vi "RT (Testing).vi"() -> ()   [LabVIEW 2015]
uses:
  <vilib>/FPGAPlugInAG/sbRIO-9626/niLvFpga_Open_sbRIO-9626.vi
  <vilib>/rvi/interface/common/dynamic/niFpgaDynamicAddResources.vi
  <vilib>/Utility/error.llb/Error Cluster From Error Code.vi
  <vilib>/rvi/errors/niLvFpgaAdjustHostInterfaceError.vi
  <vilib>/FPGAPlugInAG/Dynamic/niLvFpga_Close_Dynamic.vi
  <vilib>/rvi/interface/nirviOpenFPGA/nirviOpenFPGA.xnode
  FPGA/Bitfiles/myPAM_FPGA_FPGA(TopLevel)_6BC50j0dlkU.lvbitx
  FPGA/FPGA (Top Level).vi
  <vilib>/rvi/interface/nirviReadWriteControl/nirviReadWriteControl.xnode
  <vilib>/rvi/interface/nirviCloseFPGA/nirviCloseFPGA.xnode
  NiFpgaLv.dll
  <vilib>/rvi/interface/Simulation/niFpgaSimulationCallBeginRW.vi
panel:
  out "LINK2_DRIVE_STATUS":T1(ring)
  out "LINK1_DRIVE_STATUS":T1(ring)
  in  "LINK2_DEMAND_PWM":i16(slide) scale=-375.0..375.0
  in  "LINK1_DEMAND_PWM":i16(slide) scale=-525.0..525.0
  in  "LINK2_DRIVE_ENABLED":bool
  in  "LINK1_DRIVE_ENABLED":bool
  in  "Stop Button":bool
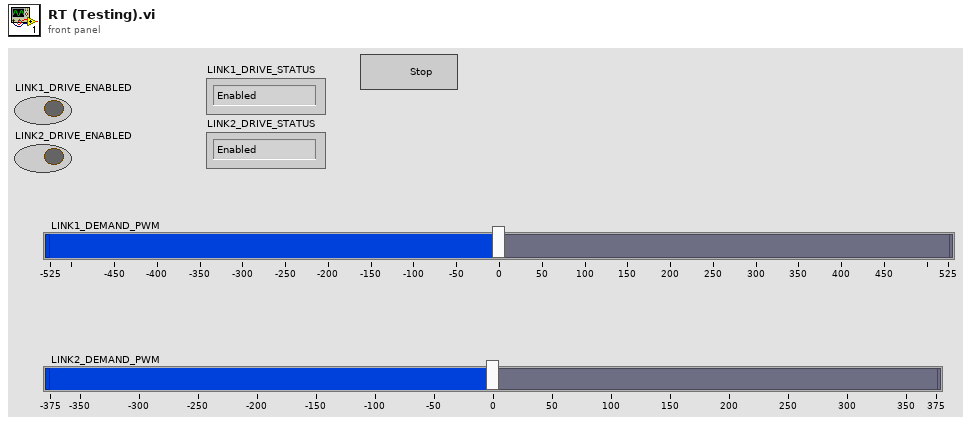
[diagram p1: front panel]
types:
  T1 = enum8{"Enabled", "Disabled", "Disabled by Drive Fault", "Disabled by Temp. Fault", "Disabled by E-Stop", "Unknown"}
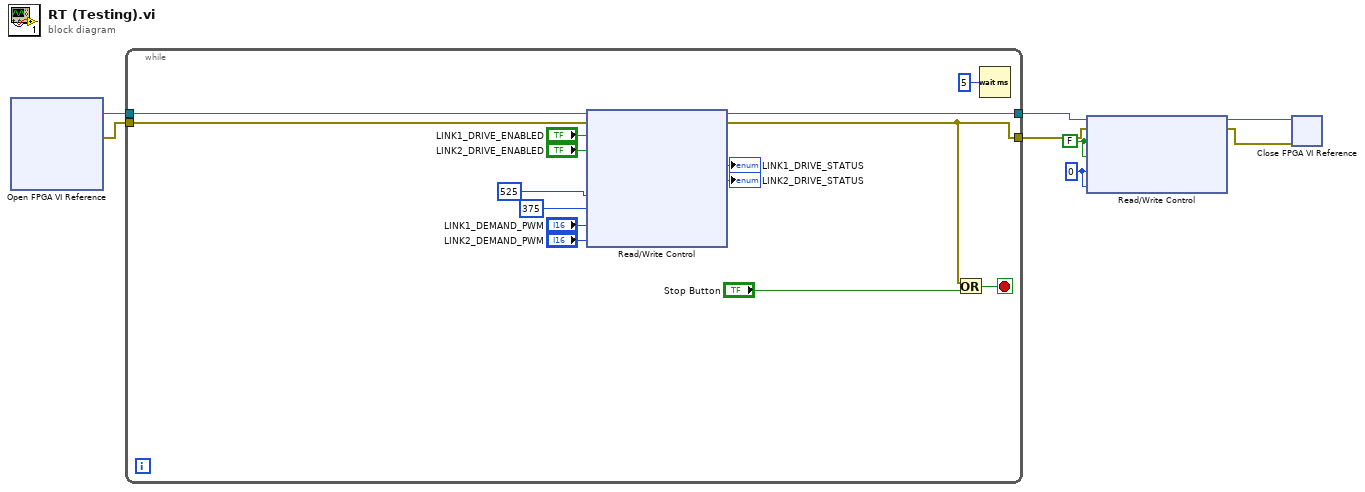
[diagram p0: block diagram]
diagram:
  w1 = i16 0 ("LINK1_DEMAND_PWM")
  w2 = FALSE ("LINK1_DRIVE_ENABLED")
  n1 = xnode "Open FPGA VI Reference"() -> ("FPGA VI Reference Out"=w8:refnum<k20>, "error out"=w7:errorcluster)  [unwired: 2 in]
  n2 = while {
    tunnel: w8 -> [w17]
    tunnel: w7 -> [w23]
    tunnel: [w22] -> w6
    tunnel: [w19] -> w5
    stop <- w18 stop-if-true
    n3 = xnode "Read/Write Control"("FPGA VI Reference In"=w17, "error in"=w23, "LINK1_DRIVE_ENABLED"="LINK1_DRIVE_ENABLED", "LINK2_DRIVE_ENABLED"="LINK2_DRIVE_ENABLED", "LINK1_PWM_MAX"=i16 525, "LINK2_PWM_MAX"=i16 375, "LINK1_DEMAND_PWM"="LINK1_DEMAND_PWM", "LINK2_DEMAND_PWM"="LINK2_DEMAND_PWM") -> ("FPGA VI Reference Out"=w22:refnum<k20>, "error out"=w19:errorcluster, "LINK1_DRIVE_STATUS"=→"LINK1_DRIVE_STATUS":T1, "LINK2_DRIVE_STATUS"=→"LINK2_DRIVE_STATUS":T1)
    n4 = Or(x=w19, y="Stop Button") -> (x .or. y?=w18:bool)
    n5 = Wait (ms)(milliseconds to wait=u32 5) -> ()  [unwired: 1 out]
  }
  n6 = xnode "Read/Write Control"("FPGA VI Reference In"=w6, "error in"=w5, "LINK1_DRIVE_ENABLED"=w2, "LINK2_DRIVE_ENABLED"=w2, "LINK1_DEMAND_PWM"=w1, "LINK2_DEMAND_PWM"=w1) -> ("FPGA VI Reference Out"=w4:refnum<k20>, "error out"=w3:errorcluster)
  n7 = xnode "Close FPGA VI Reference"("FPGA VI Reference In"=w4, "error in"=w3) -> ()  [unwired: 1 out]
